vi "ALARMS.vi"(8 "Error In":errorcluster, 10 "ALARM Input":bool[](array[boolean]), 11 "PROC OK Input":bool[](array[boolean])) -> (0 "Error Out":errorcluster, 2 "ALARM Output":bool[](array[boolean]), 3 "PROC OK Output":bool[](array[boolean]))   [LabVIEW 2023]
uses:
  procnokstringscontrol.ctl
  procnokstr.ctl
  procnokLEDScontrol.ctl
  procnokLED.ctl
  Alarmstringscontrol.ctl
  alarmstr.ctl
  AlarmLEDscontrol.ctl
  AlarmLED.ctl
  QSM - Alarms/Controls/State Machine Message.ctl
  QSM - Alarms/Controls/Message Queue Element Position.ctl
  QSM - Alarms/QSM - Alarms.lvlib
panel:
  out "ALARM LED":bool
  in  "Clear ALARMS":bool
  out "ALARMS":T1
  in  "Alarm strings":T3
  in  "MAIN Page":bool
  out "PROC NOK LED":bool
  in  "CLEAR PROCNOK":bool
  out "PROCNOK":T5
  in  "PROCNOK strings":T7
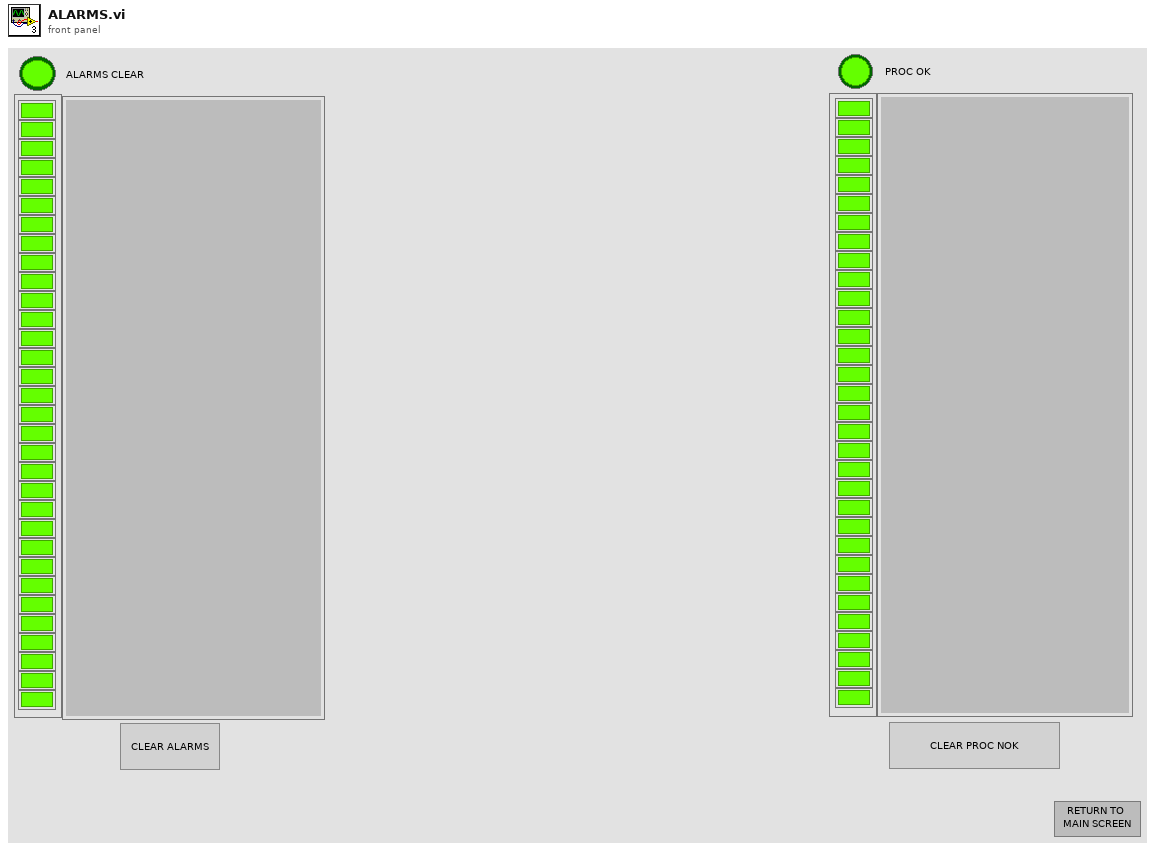
[diagram p1: front panel]
types:
  T1 = typedef "AlarmLEDscontrol.ctl" = cluster{"ALARM LIGHT":T2, "ALARM LIGHT 2":T2, "ALARM LIGHT 3":T2, "ALARM LIGHT 4":T2, "ALARM LIGHT 5":T2, "ALARM LIGHT 6":T2, "ALARM LIGHT 7":T2, "ALARM LIGHT 8":T2, "ALARM LIGHT 9":T2, "ALARM LIGHT 10":T2, "ALARM LIGHT 11":T2, "ALARM LIGHT 12":T2, "ALARM LIGHT 13":T2, "ALARM LIGHT 14":T2, "ALARM LIGHT 15":T2, "ALARM LIGHT 16":T2, "ALARM LIGHT 17":T2, "ALARM LIGHT 18":T2, "ALARM LIGHT 19":T2, "ALARM LIGHT 20":T2, "ALARM LIGHT 21":T2, "ALARM LIGHT 22":T2, "ALARM LIGHT 23":T2, "ALARM LIGHT 24":T2, "ALARM LIGHT 25":T2, "ALARM LIGHT 26":T2, "ALARM LIGHT 27":T2, "ALARM LIGHT 28":T2, "ALARM LIGHT 29":T2, "ALARM LIGHT 30":T2, "ALARM LIGHT 31":T2, "ALARM LIGHT 32":T2}
  T2 = typedef "AlarmLED.ctl" = bool
  T3 = typedef "Alarmstringscontrol.ctl" = cluster{"Alarm str":T4, "Alarm str 2":T4, "Alarm str 3":T4, "Alarm str 4":T4, "Alarm str 5":T4, "Alarm str 6":T4, "Alarm str 7":T4, "Alarm str 8":T4, "Alarm str 9":T4, "Alarm str 10":T4, "Alarm str 11":T4, "Alarm str 12":T4, "Alarm str 13":T4, "Alarm str 14":T4, "Alarm str 15":T4, "Alarm str 16":T4, "Alarm str 17":T4, "Alarm str 18":T4, "Alarm str 19":T4, "Alarm str 20":T4, "Alarm str 21":T4, "Alarm str 22":T4, "Alarm str 23":T4, "Alarm str 24":T4, "Alarm str 25":T4, "Alarm str 26":T4, "Alarm str 27":T4, "Alarm str 28":T4, "Alarm str 29":T4, "Alarm str 30":T4, "Alarm str 31":T4, "Alarm str 32":T4}
  T4 = typedef "alarmstr.ctl" = string
  T5 = typedef "procnokLEDScontrol.ctl" = cluster{"PROCNOK":T6, "PROCNOK 2":T6, "PROCNOK 3":T6, "PROCNOK 4":T6, "PROCNOK 5":T6, "PROCNOK 6":T6, "PROCNOK 7":T6, "PROCNOK 8":T6, "PROCNOK 9":T6, "PROCNOK 10":T6, "PROCNOK 11":T6, "PROCNOK 12":T6, "PROCNOK 13":T6, "PROCNOK 14":T6, "PROCNOK 15":T6, "PROCNOK 16":T6, "PROCNOK 17":T6, "PROCNOK 18":T6, "PROCNOK 19":T6, "PROCNOK 20":T6, "PROCNOK 21":T6, "PROCNOK 22":T6, "PROCNOK 23":T6, "PROCNOK 24":T6, "PROCNOK 25":T6, "PROCNOK 26":T6, "PROCNOK 27":T6, "PROCNOK 28":T6, "PROCNOK 29":T6, "PROCNOK 30":T6, "PROCNOK 31":T6, "PROCNOK 32":T6}
  T6 = typedef "procnokLED.ctl" = bool
  T7 = typedef "procnokstringscontrol.ctl" = cluster{"PROCNOKSTR":T8, "PROCNOKSTR 2":T8, "PROCNOKSTR 3":T8, "PROCNOKSTR 4":T8, "PROCNOKSTR 5":T8, "PROCNOKSTR 6":T8, "PROCNOKSTR 7":T8, "PROCNOKSTR 8":T8, "PROCNOKSTR 9":T8, "PROCNOKSTR 10":T8, "PROCNOKSTR 11":T8, "PROCNOKSTR 12":T8, "PROCNOKSTR 13":T8, "PROCNOKSTR 14":T8, "PROCNOKSTR 15":T8, "PROCNOKSTR 16":T8, "PROCNOKSTR 17":T8, "PROCNOKSTR 18":T8, "PROCNOKSTR 19":T8, "PROCNOKSTR 20":T8, "PROCNOKSTR 21":T8, "PROCNOKSTR 22":T8, "PROCNOKSTR 23":T8, "PROCNOKSTR 24":T8, "PROCNOKSTR 25":T8, "PROCNOKSTR 26":T8, "PROCNOKSTR 27":T8, "PROCNOKSTR 28":T8, "PROCNOKSTR 29":T8, "PROCNOKSTR 30":T8, "PROCNOKSTR 31":T8, "PROCNOKSTR 32":T8}
  T8 = typedef "procnokstr.ctl" = string
  T9 = typedef "QSM - Alarms.lvlib/State Machine Message.ctl" = enum16{"Initialize", "PROC OK Change", "CLEAR PROC NOK", "ALARM SET", "CLEAR ALARMS", "Handle Error", "Exit"}
  T10 = typedef "QSM - Alarms.lvlib/Message Queue Element Position.ctl" = enum16{"Front", "Back"}
  T11 = cluster{"Value[0]":bool, "Value[1]":bool, "Value[2]":bool, "Value[3]":bool, "Value[4]":bool, "Value[5]":bool, "Value[6]":bool, "Value[7]":bool, "Value[8]":bool, "Value[9]":bool, "Value[10]":bool, "Value[11]":bool, "Value[12]":bool, "Value[13]":bool, "Value[14]":bool, "Value[15]":bool, "Value[16]":bool, "Value[17]":bool, "Value[18]":bool, "Value[19]":bool, "Value[20]":bool, "Value[21]":bool, "Value[22]":bool, "Value[23]":bool, "Value[24]":bool, "Value[25]":bool, "Value[26]":bool, "Value[27]":bool, "Value[28]":bool, "Value[29]":bool, "Value[30]":bool, "Value[31]":bool}
  T12 = cluster{"[0]":bool, "[1]":bool, "[2]":bool, "[3]":bool, "[4]":bool, "[5]":bool, "[6]":bool, "[7]":bool, "[8]":bool, "[9]":bool, "[10]":bool, "[11]":bool, "[12]":bool, "[13]":bool, "[14]":bool, "[15]":bool, "[16]":bool, "[17]":bool, "[18]":bool, "[19]":bool, "[20]":bool, "[21]":bool, "[22]":bool, "[23]":bool, "[24]":bool, "[25]":bool, "[26]":bool, "[27]":bool, "[28]":bool, "[29]":bool, "[30]":bool, "[31]":bool}
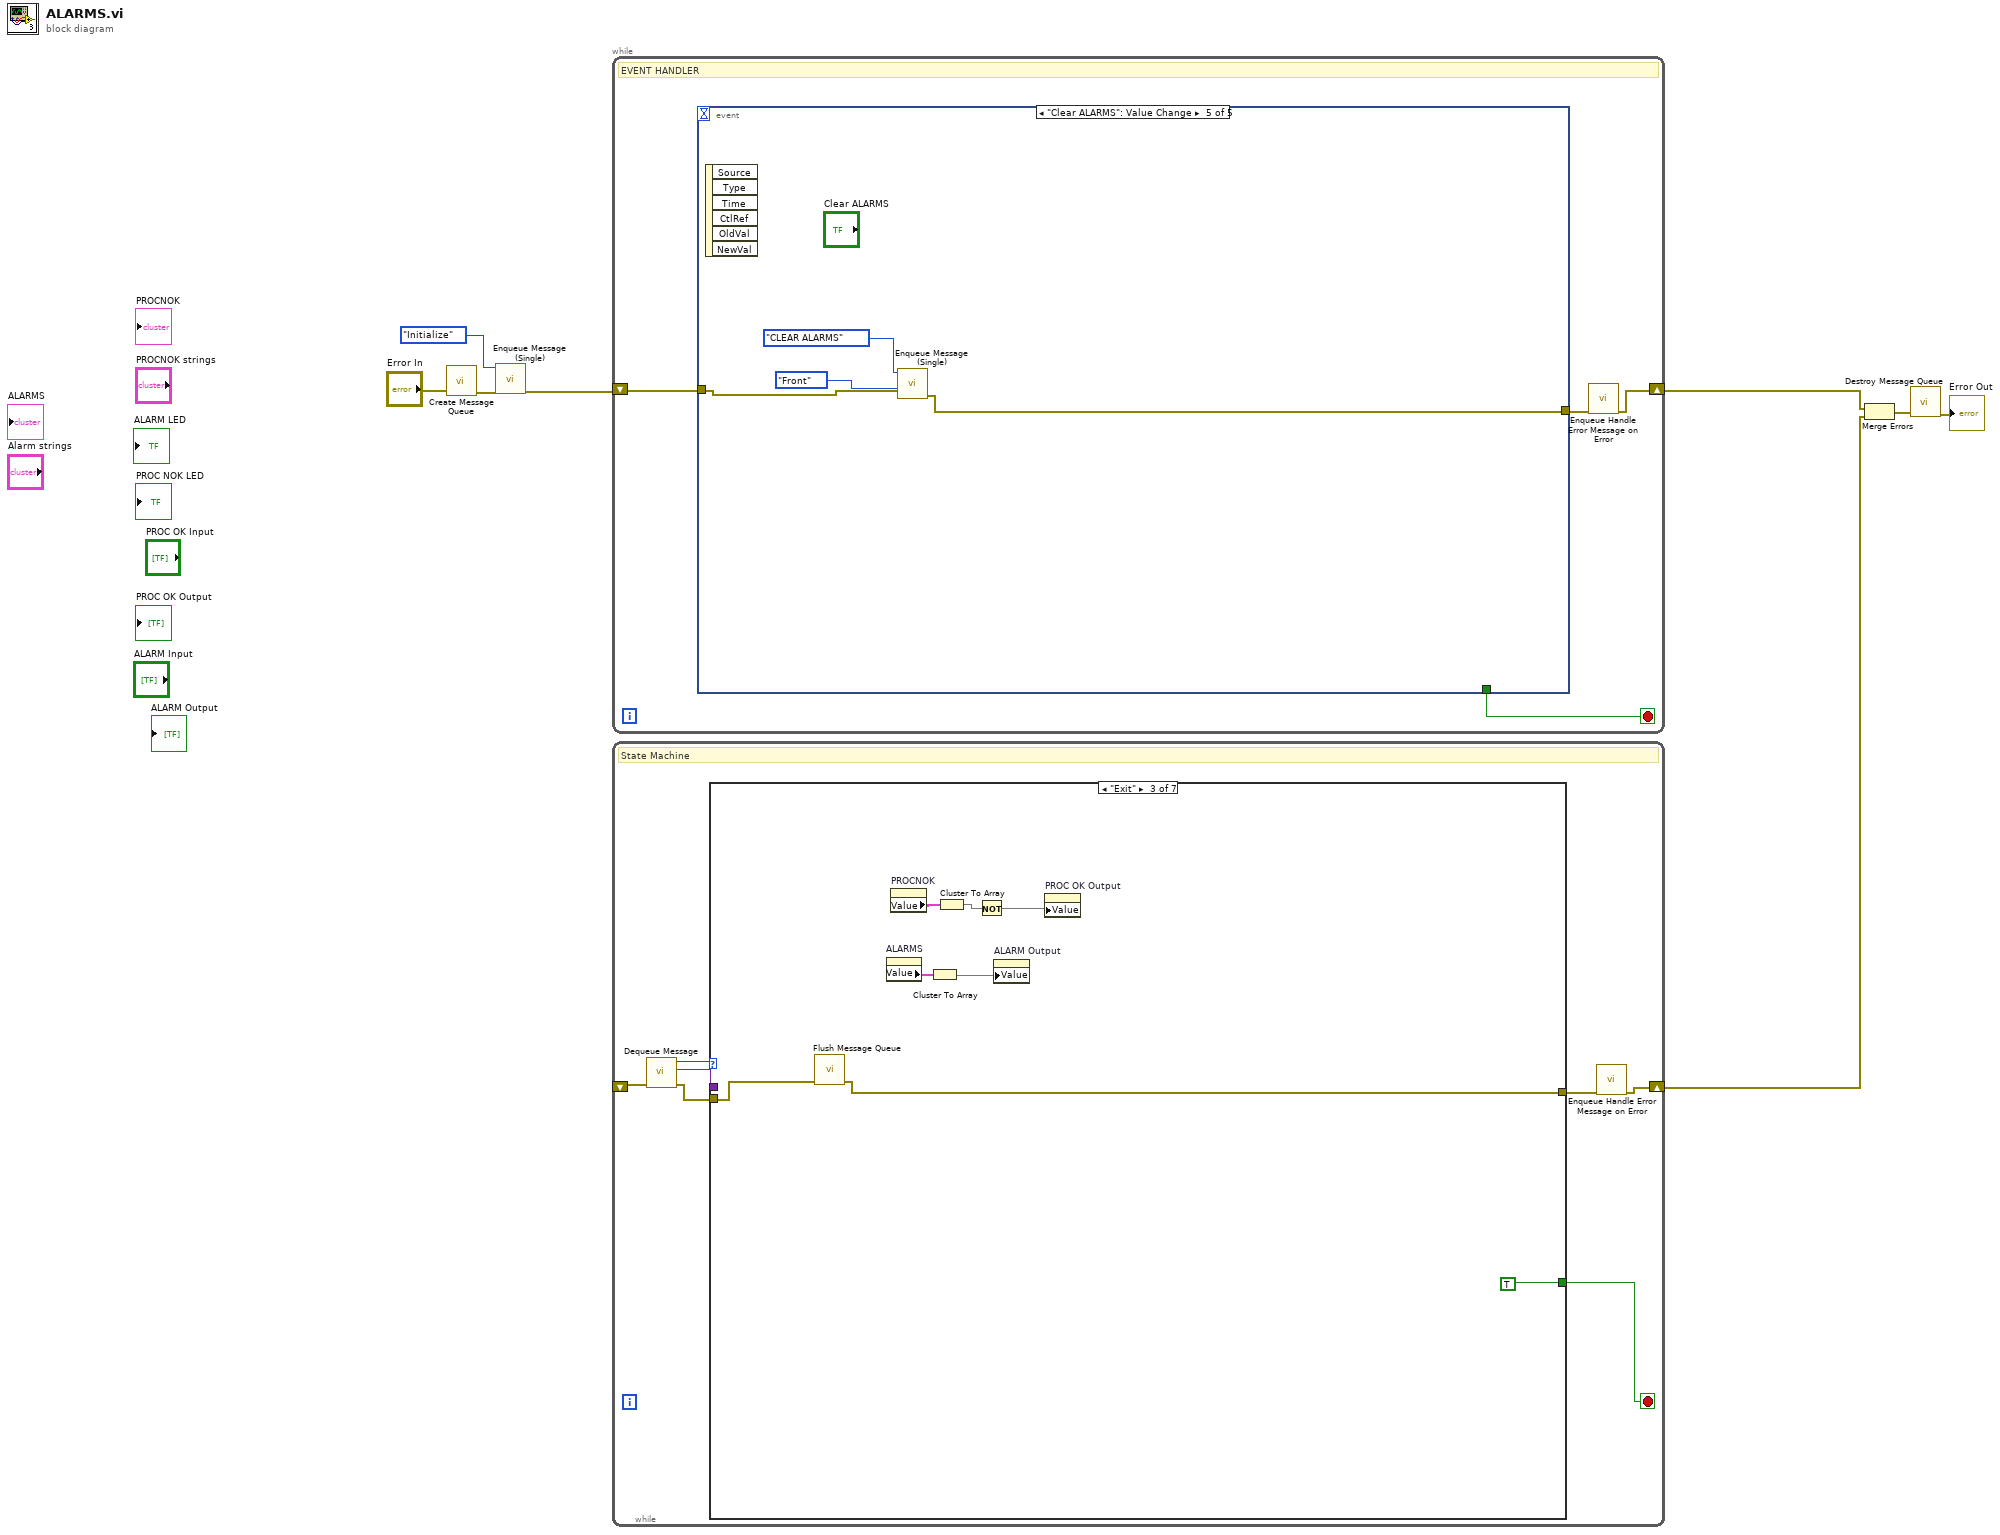
[diagram p0: block diagram]
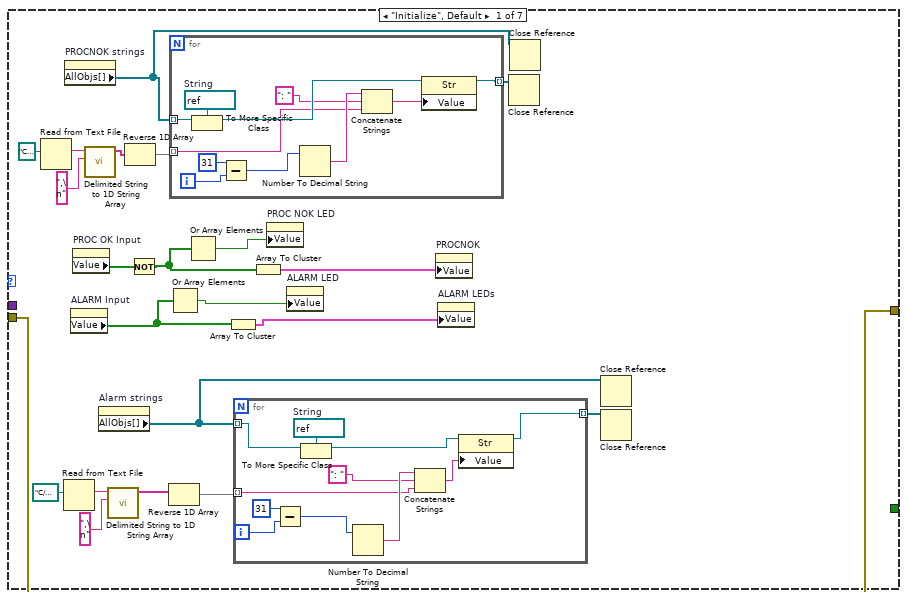
[diagram p2: hidden frame]
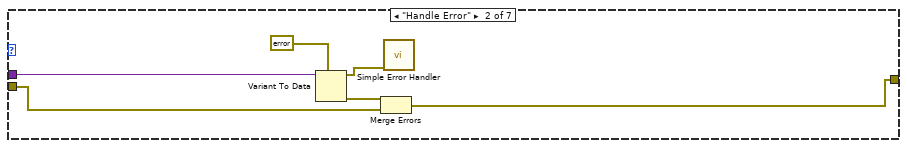
[diagram p3: hidden frame]
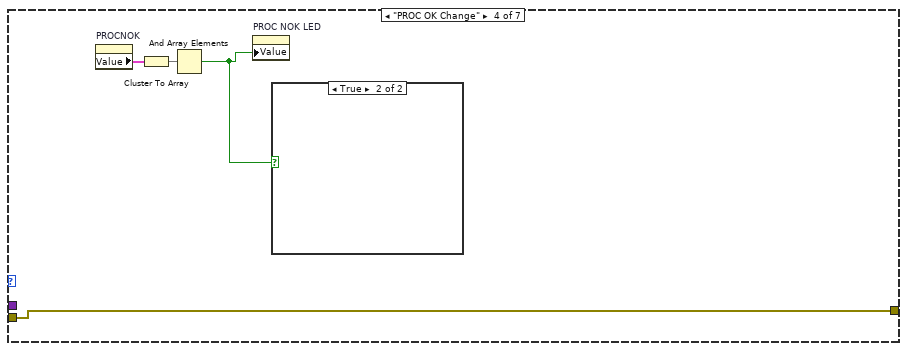
[diagram p4: hidden frame]
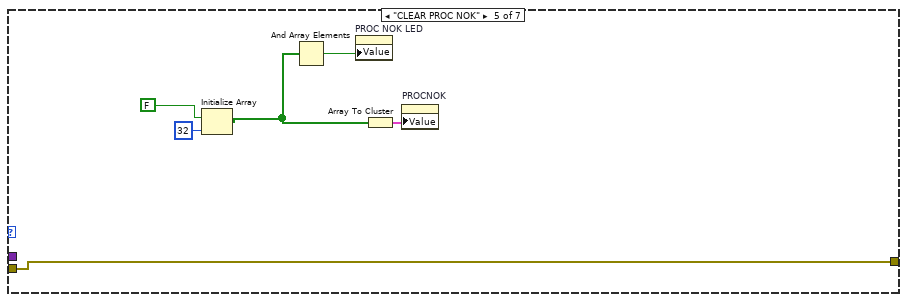
[diagram p6: hidden frame]
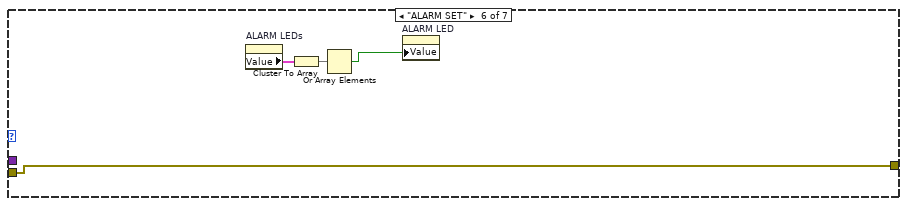
[diagram p7: hidden frame]
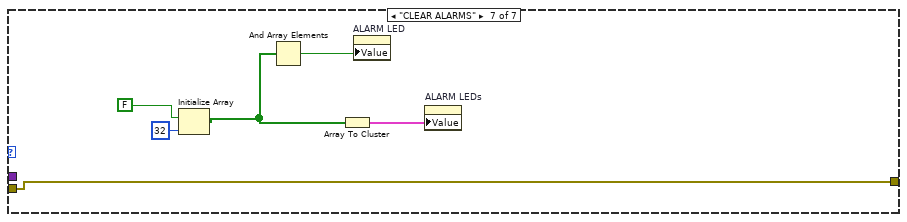
[diagram p8: hidden frame]
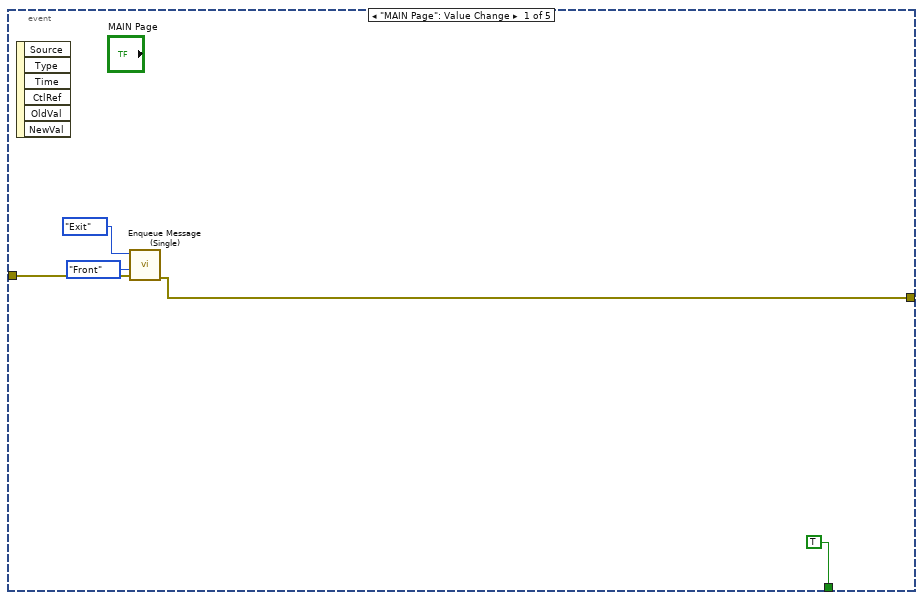
[diagram p9: hidden frame]
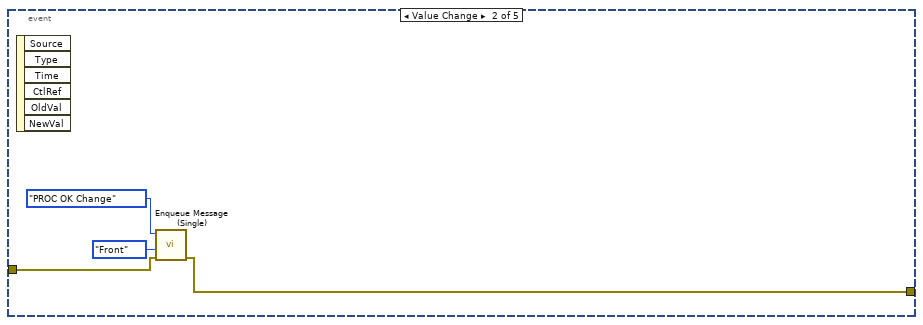
[diagram p10: hidden frame]
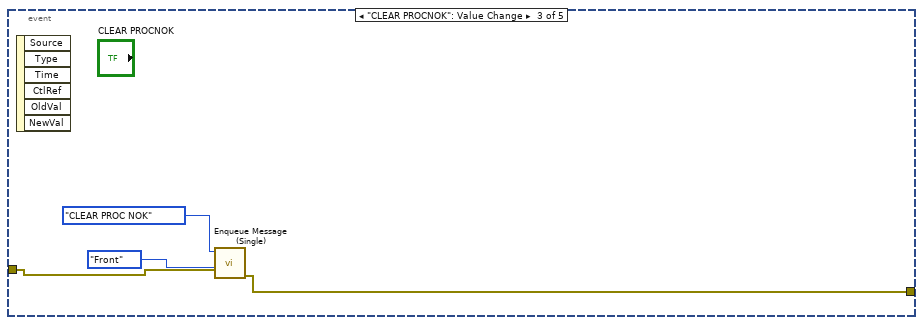
[diagram p11: hidden frame]
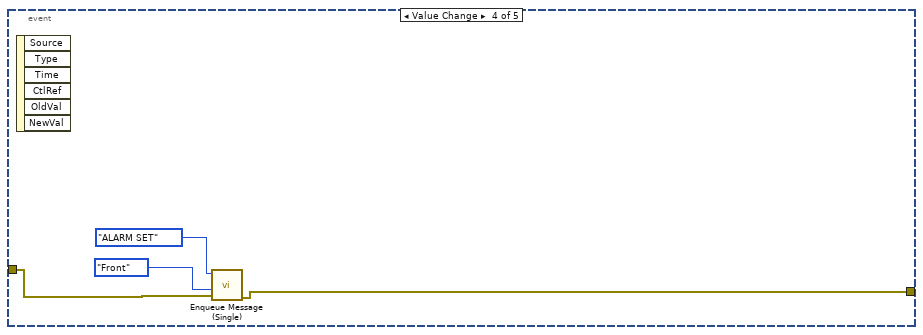
[diagram p12: hidden frame]
diagram:
  n1 = call "Create Message Queue.vi"("Error In"="Error In") -> ("Error Out"=w7:errorcluster)  [unwired: 10 in]
  n2 = call "Enqueue Message (Single).vi"("Error In"=w7, "State Machine Message"=State_Machine_Message."Initialize") -> ("Error Out"=w6:errorcluster)  [unwired: 9 in]
  n3 = while {
    shift-right: [w11] -> w2
    shift-left: w6 -> [w12]
    stop <- w9 stop-if-true
    # "EVENT HANDLER"
    n4 = event shown="[4] \"Clear ALARMS\": Value Change" {
      selector: _ -> [_ _ _ _ _]
      dyn-events: _ -> [_ _ _ _ _]
      timeout: _ -> [_ _ _ _ _]
      tunnel: w12 -> [w17 w19 w23 w27 w31]
      tunnel: [w14 w18 w22 w26 w30] -> w10
      tunnel: [TRUE _ _ _ _] -> w9
      event "MAIN Page": Value Change {
        n5 = event-data() -> ()  [unwired: 1 in, 6 out]
        n6 = call "Enqueue Message (Single).vi"("Error In"=w17, "Message Position"=Message_Queue_Element_Position."Front", "State Machine Message"=State_Machine_Message."Exit") -> ("Error Out"=w14:errorcluster)  [unwired: 8 in]
      }
      event Value Change {
        n7 = event-data() -> ()  [unwired: 1 in, 6 out]
        n8 = call "Enqueue Message (Single).vi"("Error In"=w19, "Message Position"=Message_Queue_Element_Position."Front", "State Machine Message"=State_Machine_Message."PROC OK Change") -> ("Error Out"=w18:errorcluster)  [unwired: 8 in]
      }
      event "CLEAR PROCNOK": Value Change {
        n9 = event-data() -> ()  [unwired: 1 in, 6 out]
        n10 = call "Enqueue Message (Single).vi"("Error In"=w23, "Message Position"=Message_Queue_Element_Position."Front", "State Machine Message"=State_Machine_Message."CLEAR PROC NOK") -> ("Error Out"=w22:errorcluster)  [unwired: 8 in]
      }
      event Value Change {
        n11 = event-data() -> ()  [unwired: 1 in, 6 out]
        n12 = call "Enqueue Message (Single).vi"("Error In"=w27, "Message Position"=Message_Queue_Element_Position."Front", "State Machine Message"=State_Machine_Message."ALARM SET") -> ("Error Out"=w26:errorcluster)  [unwired: 8 in]
      }
      event "Clear ALARMS": Value Change {
        n13 = event-data() -> ()  [unwired: 1 in, 6 out]
        n14 = call "Enqueue Message (Single).vi"("Error In"=w31, "Message Position"=Message_Queue_Element_Position."Front", "State Machine Message"=State_Machine_Message."CLEAR ALARMS") -> ("Error Out"=w30:errorcluster)  [unwired: 8 in]
      }
    }
    n15 = call "Enqueue Handle Error Message on Error.vi"("Error In"=w10) -> ("Error Out"=w11:errorcluster)  [unwired: 10 in]
  }
  n16 = while {
    shift-right: [w40] -> w1
    shift-left: _ -> [w39]
    stop <- w34 stop-if-true
    # "State Machine"
    n17 = call "Dequeue Message.vi"("Error In"=w39) -> ("Error Out"=w37:errorcluster, "Data"=w35:variant, "State Machine Message"=w38:T9)  [unwired: 8 in]
    n18 = case shown="\"Exit\"" w38 {
      tunnel: w37 -> [w62 w87 w98 w99 w108 w109 w113]
      tunnel: [w62 w85 w97 w99 w108 w109 w113] -> w36
      tunnel: w35 -> [_ w86 _ _ _ _ _]
      tunnel: [_ _ TRUE _ _ _ _] -> w34
      frame "Initialize", Default {
        n19 = Read from Text File(file (use dialog)=path "C:/Users/Public/Documents/Grid2093/ALARMS/PROCNOK.txt") -> (text=w59:string)  [unwired: 3 in, 3 out]
        n20 = Read from Text File(file (use dialog)=path "C:/Users/Public/Documents/Grid2093/ALARMS/ALARMS.txt") -> (text=w50:string)  [unwired: 3 in, 3 out]
        n21 = property on="PROCNOK strings" class="Clust (strict)"() -> ("AllObjs[]"=w61:refnum<vi>[])  [unwired: 2 in, 2 out]
        n22 = property on="ALARM Input" class="Arr (strict)"() -> ("Value"=w47:bool[])  [unwired: 2 in, 2 out]
        n23 = property on="PROC OK Input" class="Arr (strict)"() -> ("Value"=w55:bool[])  [unwired: 2 in, 2 out]
        n24 = call <vilib>:"Delimited String to 1D String Array.vi"("delimiter"=",\n", "delimited string"=w59) -> ("string array"=w44:string[])  [unwired: 9 in]
        n25 = property on="Alarm strings" class="Clust (strict)"() -> ("AllObjs[]"=w49:refnum<vi>[])  [unwired: 2 in, 2 out]
        n26 = call <vilib>:"Delimited String to 1D String Array.vi"("delimiter"=",\n", "delimited string"=w50) -> ("string array"=w42:string[])  [unwired: 9 in]
        n27 = Reverse 1D Array(array=w44) -> (reversed array=w43:string[])
        n28 = Not(x=w55) -> (.not. x?=w53:bool[])
        n29 = Reverse 1D Array(array=w42) -> (reversed array=w41:string[])
        n30 = for {
          tunnel: [w82] -> w60 mode=indexing
          tunnel: w43 -> [w78] mode=indexing
          tunnel: w61 -> [w77] mode=indexing
          i -> [w75]
          w84 = refnum<vi> refnum  # String
          n31 = To More Specific Class(target class=w84, reference=w77) -> (specific class reference=w83:refnum<vi>)  [unwired: 1 in, 1 out]
          n32 = Subtract(x=31, y=w75) -> (x-y=w74:i32)
          n33 = Number To Decimal String(number=w74) -> (decimal integer string=w80:string)  [unwired: 1 in]
          n34 = Concatenate Strings(w80, ": " ("string"), w78) -> (w81:string)
          n35 = property class="Str"(reference=w83, "Value"=w81) -> (reference out=w82:refnum<vi>)  [unwired: 1 in, 1 out]
        }
        n36 = Or Array Elements(Boolean array=w47) -> (logical OR=w45:bool)
        n37 = Or Array Elements(Boolean array=w53) -> (logical OR=w54:bool)
        n38 = Array To Cluster(array=w47) -> (cluster=w46:T11)
        n39 = for {
          tunnel: w41 -> [w69] mode=indexing
          tunnel: w49 -> [w73] mode=indexing
          tunnel: [w66] -> w48 mode=indexing
          i -> [w64]
          w72 = refnum<vi> refnum  # String
          n40 = Subtract(x=31, y=w64) -> (x-y=w63:i32)
          n41 = To More Specific Class(target class=w72, reference=w73) -> (specific class reference=w67:refnum<vi>)  [unwired: 1 in, 1 out]
          n42 = Number To Decimal String(number=w63) -> (decimal integer string=w71:string)  [unwired: 1 in]
          n43 = Concatenate Strings(w71, ": " ("string"), w69) -> (w68:string)
          n44 = property class="Str"(reference=w67, "Value"=w68) -> (reference out=w66:refnum<vi>)  [unwired: 1 in, 1 out]
        }
        n45 = Array To Cluster(array=w53) -> (cluster=w56:T12)
        n46 = property on="PROC NOK LED" class="Bool (strict)"("Value"=w54) -> ()  [unwired: 2 in, 2 out]
        n47 = property on="ALARM LED" class="Bool (strict)"("Value"=w45) -> ()  [unwired: 2 in, 2 out]
        n48 = property on="PROCNOK" class="Clust (strict)"("Value"=w56) -> ()  [unwired: 2 in, 2 out]
        n49 = property on="ALARM LEDs" class="Clust (strict)"("Value"=w46) -> ()  [unwired: 2 in, 2 out]
        n50 = Close Reference(reference=w60) -> ()  [unwired: 1 in, 1 out]
        n51 = Close Reference(reference=w61) -> ()  [unwired: 1 in, 1 out]
        n52 = Close Reference(reference=w49) -> ()  [unwired: 1 in, 1 out]
        n53 = Close Reference(reference=w48) -> ()  [unwired: 1 in, 1 out]
      }
      frame "Handle Error" {
        n54 = Variant To Data(type=errorcluster {"status"=FALSE, "code"=0, "source"=""} ("Error In"), Variant=w86) -> (data=w88:errorcluster, error out=w89:errorcluster)  [unwired: 1 in]
        n55 = Merge Errors(w89, w87) -> (w85:errorcluster)
        n56 = call <vilib>:"Simple Error Handler.vi"("error in (no error)"=w88) -> ()  [unwired: 4 in, 5 out]
      }
      frame "Exit" {
        n57 = call "Flush Message Queue.vi"("Error In"=w98) -> ("Error Out"=w97:errorcluster)  [unwired: 9 in, 1 out]
        n58 = property on="ALARMS" class="Clust (strict)"() -> ("Value"=w92:T1)  [unwired: 2 in, 2 out]
        n59 = property on="PROCNOK" class="Clust (strict)"() -> ("Value"=w94:T5)  [unwired: 2 in, 2 out]
        n60 = Cluster To Array(cluster=w92) -> (array=w91:T2[])
        n61 = Cluster To Array(cluster=w94) -> (array=w93:T6[])
        n62 = Not(x=w93) -> (.not. x?=w95:T6[])
        n63 = property on="ALARM Output" class="Arr (strict)"("Value"=w91) -> ()  [unwired: 2 in, 2 out]
        n64 = property on="PROC OK Output" class="Arr (strict)"("Value"=w95) -> ()  [unwired: 2 in, 2 out]
      }
      frame "PROC OK Change" {
        n65 = property on="PROCNOK" class="Clust (strict)"() -> ("Value"=w102:T5)  [unwired: 2 in, 2 out]
        n66 = Cluster To Array(cluster=w102) -> (array=w101:T6[])
        n67 = And Array Elements(Boolean array=w101) -> (logical AND=w100:bool)
        n68 = property on="PROC NOK LED" class="Bool (strict)"("Value"=w100) -> ()  [unwired: 2 in, 2 out]
        n69 = case shown="True" w100 {
          frame False {
          }
          frame True {
          }
        }
      }
      frame "CLEAR PROC NOK" {
        n70 = Initialize Array(FALSE, 32 ("dimension size")) -> (w104:bool[])
        n71 = And Array Elements(Boolean array=w104) -> (logical AND=w103:bool)
        n72 = property on="PROC NOK LED" class="Bool (strict)"("Value"=w103) -> ()  [unwired: 2 in, 2 out]
        n73 = Array To Cluster(array=w104) -> (cluster=w107:T12)
        n74 = property on="PROCNOK" class="Clust (strict)"("Value"=w107) -> ()  [unwired: 2 in, 2 out]
      }
      frame "ALARM SET" {
        n75 = property on="ALARM LEDs" class="Clust (strict)"() -> ("Value"=w112:T1)  [unwired: 2 in, 2 out]
        n76 = Cluster To Array(cluster=w112) -> (array=w111:T2[])
        n77 = Or Array Elements(Boolean array=w111) -> (logical OR=w110:bool)
        n78 = property on="ALARM LED" class="Bool (strict)"("Value"=w110) -> ()  [unwired: 2 in, 2 out]
      }
      frame "CLEAR ALARMS" {
        n79 = Initialize Array(FALSE, 32 ("dimension size")) -> (w115:bool[])
        n80 = And Array Elements(Boolean array=w115) -> (logical AND=w114:bool)
        n81 = Array To Cluster(array=w115) -> (cluster=w118:T12)
        n82 = property on="ALARM LED" class="Bool (strict)"("Value"=w114) -> ()  [unwired: 2 in, 2 out]
        n83 = property on="ALARM LEDs" class="Clust (strict)"("Value"=w118) -> ()  [unwired: 2 in, 2 out]
      }
    }
    n84 = call "Enqueue Handle Error Message on Error.vi"("Error In"=w36) -> ("Error Out"=w40:errorcluster)  [unwired: 10 in]
  }
  n85 = Merge Errors(w2, w1) -> (w3:errorcluster)
  n86 = call "Destroy Message Queue.vi"("Error In"=w3) -> ("Error Out"=→"Error Out":errorcluster)  [unwired: 10 in]
